vi "_CSM - Read File Logger Configuration - v1.0.vi"(5 "Section Name(\"FileLogger\")":string="FileLogger", 7 "error in (no error)":errorcluster) -> (1 "error out":errorcluster, 3 "FileLogger Configuration-v1":T1={"Enable"=TRUE, "Limit"={"FileSize"=10000000, "FileNum"=2}, "Timestamp.Format"="%<%Y/%m/%d %H:%M:%S%3u>T", "AutoExit"=FALSE} {"Limit"."FileSize" format="%.0p"})   [LabVIEW 2017, in "INI-Static-Variable-Support.lvlib"]
uses:
  INI-Static-Variable-Support.lvlib
  _fgv-oper.ctl
  global-csm-ini-db-change-flag.vi
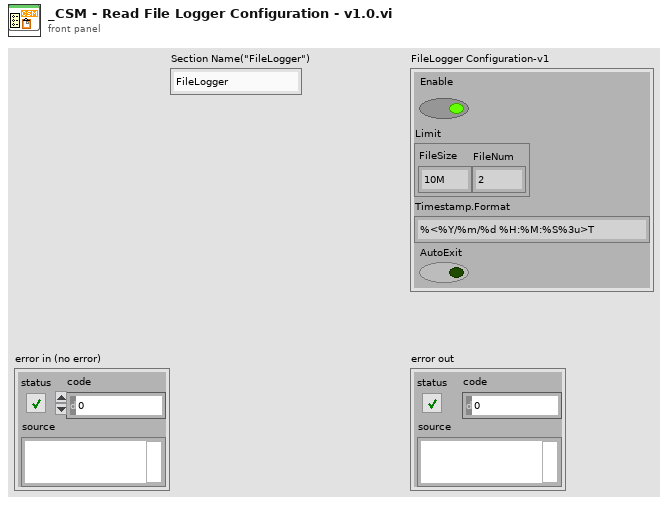
[diagram p1: front panel]
types:
  T1 = cluster{"Enable":bool, "Limit":cluster{"FileSize":i64, "FileNum":i32}, "Timestamp.Format":string, "AutoExit":bool}
  T2 = typedef "INI-Static-Variable-Support.lvlib/_fgv-oper.ctl" = enum16{"Read", "Write", "Sync", "Sessions", "List Keys", "Load", "List Files", "List Variables", "List Permanent Variables", "Mark Temp Variable as Permenent", "unload", "INIConfig(Memory)", "Reset", "Restore Variable Value"}
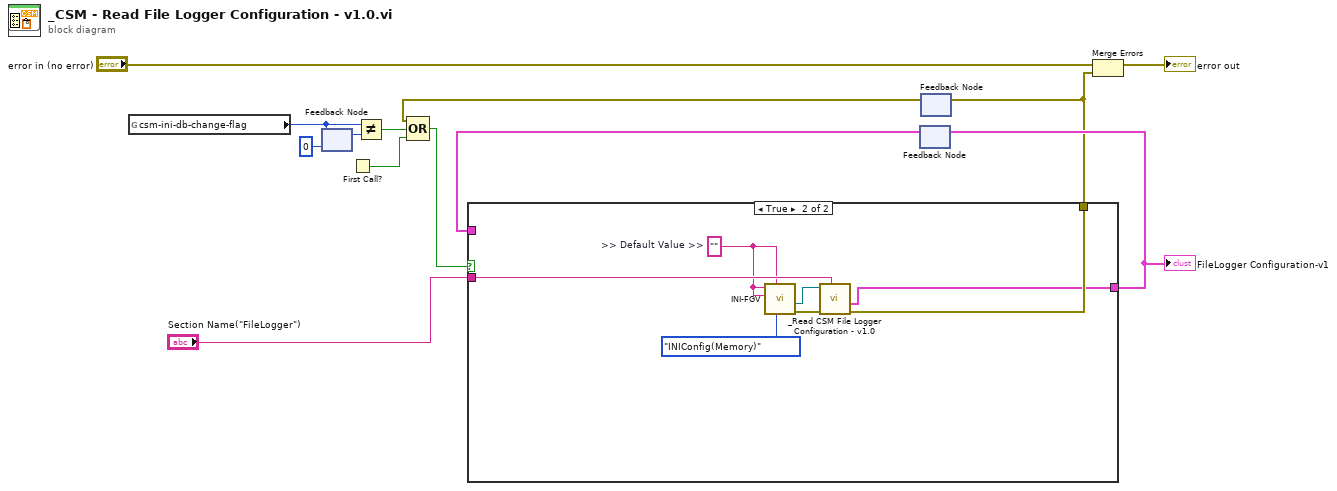
[diagram p0: block diagram]
diagram:
  n1 = global read "global-csm-ini-db-change-flag.vi" "csm-ini-db-change-flag"() -> (w11:u64)
  n2 = feedback #1(u64 0 ("csm-ini-db-change-flag")) -> (w10:u64)
  n3 = feedback-in #1(w11) -> ()
  n4 = First Call?() -> (First Call?: T/F=w1:bool)
  n5 = Not Equal?(x=w11, y=w10) -> (x != y?=w9:bool)
  n6 = feedback #2() -> (w7:T1)  [unwired: 1 in]
  n7 = feedback #3() -> (w5:errorcluster)  [unwired: 1 in]
  n8 = Compound Arithmetic op=OR(w5, w9, w1) -> (w4:bool)
  n9 = case shown="True" w4 {
    tunnel: [_ w19] -> w6
    tunnel: [w14 w18] -> w8
    tunnel: w7 -> [w14 _]
    tunnel: "Section Name(\"FileLogger\")" -> [_ w16]
    frame False {
    }
    frame True {
      w15 = ""  # >> Default Value >>
      n10 = call "INI-FGV.vi"("Enum"=_fgv-oper."INIConfig(Memory)", "Prefered Section"=w15, ">> Default Value >>"=w15, ">> Variable Name >>"=w15) -> ("error out"=w20:errorcluster, "INIConfig"=w17:refnum<class "LabVIEW-Config.lvclass">)  [unwired: 4 in, 2 out]
      n11 = call "_Read CSM File Logger Configuration - v1.0.vi"("Section Name"=w16, "error in (no error)"=w20, "LabVIEW-Config.lvlib:LabVIEW-Config.lvclass"=w17) -> ("error out"=w19:errorcluster, "FileLogger Configuration-v1"=w18:T1)  [unwired: 6 in, 1 out]
    }
  }
  "FileLogger Configuration-v1" <- w8
  n12 = feedback-in #2(w8) -> ()
  n13 = feedback-in #3(w6) -> ()
  n14 = Merge Errors("error in (no error)", w6) -> (→"error out":errorcluster)
